vi "Clusterwitharraydouble.vi"(1 "Cluster In":cluster{"Array In":dbl[], "Numeric Input":dbl} {"Numeric Input" format="%.2f"; "Array In" format="%.2f"}, 2 "Base":dbl format="%.2f") -> (0 "Cluster Out":cluster{"Array Out":dbl[], "Numeric Output":dbl} {"Numeric Output" format="%.2f"; "Array Out" format="%.2f"})   [LabVIEW 2011]
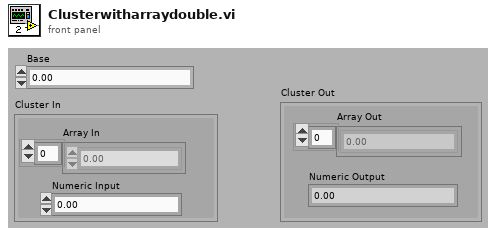
[diagram p1: front panel]
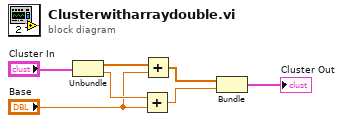
[diagram p0: block diagram]
diagram:
  n1 = Unbundle("Cluster In") -> ("Array In"=w7:dbl[], "Numeric Input"=w6:dbl)
  n2 = Add(x=w6, y="Base") -> (x+y=w4:dbl)
  n3 = Add(x=w7, y="Base") -> (x+y=w5:dbl[])
  n4 = Bundle(w5, w4) -> (→"Cluster Out":cluster{dbl[], dbl})  [unwired: 1 out]
